vi "Link Blob To Lines.vi"(1 "Lines Calibrated":T3(array[cluster]), 2 "Blob Array":T2(array[cluster])) -> (0 "TargetArray":T1(array[cluster]))   [LabVIEW 2011]
uses:
  <vilib>/Analysis/geometry.llb/Point in Polygon Position.ctl
  <vilib>/Analysis/geometry.llb/Point in Polygon (Scalar).vi
  <vilib>/vision/NI_Vision_Development_Module.lvlib
  <vilib>/Analysis/NI_AAL_Geometry.lvlib
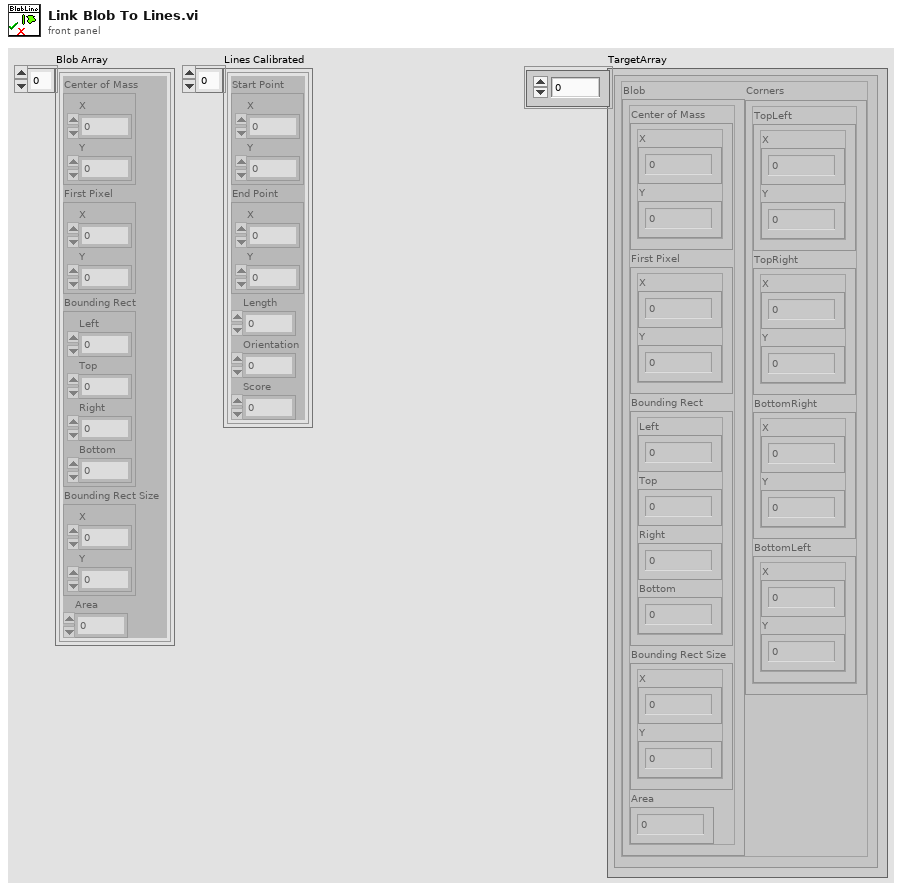
[diagram p1: front panel]
types:
  T1 = cluster{"Blob":cluster{"Center of Mass":cluster{"X":dbl, "Y":dbl}, "First Pixel":cluster{"X":dbl, "Y":dbl}, "Bounding Rect":cluster{"Left":dbl, "Top":dbl, "Right":dbl, "Bottom":dbl}, "Bounding Rect Size":cluster{"X":dbl, "Y":dbl}, "Area":dbl}, "Corners":cluster{"TopLeft":cluster{"X":dbl, "Y":dbl}, "TopRight":cluster{"X":dbl, "Y":dbl}, "BottomRight":cluster{"X":dbl, "Y":dbl}, "BottomLeft":cluster{"X":dbl, "Y":dbl}}}[]
  T2 = cluster{"Center of Mass":cluster{"X":dbl, "Y":dbl}, "First Pixel":cluster{"X":dbl, "Y":dbl}, "Bounding Rect":cluster{"Left":dbl, "Top":dbl, "Right":dbl, "Bottom":dbl}, "Bounding Rect Size":cluster{"X":dbl, "Y":dbl}, "Area":dbl}[]
  T3 = cluster{"Start Point":cluster{"X":sgl, "Y":sgl}, "End Point":cluster{"X":sgl, "Y":sgl}, "Length":dbl, "Orientation":dbl, "Score":dbl}[]
  T4 = cluster{"Blob":cluster{"Center of Mass":cluster{"X":dbl, "Y":dbl}, "First Pixel":cluster{"X":dbl, "Y":dbl}, "Bounding Rect":cluster{"Left":dbl, "Top":dbl, "Right":dbl, "Bottom":dbl}, "Bounding Rect Size":cluster{"X":dbl, "Y":dbl}, "Area":dbl}, "Lines":cluster{"Start Point":cluster{"X":sgl, "Y":sgl}, "End Point":cluster{"X":sgl, "Y":sgl}, "Length":dbl, "Orientation":dbl, "Score":dbl}[]}[]
  T5 = cluster{"Blob":cluster{"Center of Mass":cluster{"X":dbl, "Y":dbl}, "First Pixel":cluster{"X":dbl, "Y":dbl}, "Bounding Rect":cluster{"Left":dbl, "Top":dbl, "Right":dbl, "Bottom":dbl}, "Bounding Rect Size":cluster{"X":dbl, "Y":dbl}, "Area":dbl}, "Lines":cluster{"Start Point":cluster{"X":sgl, "Y":sgl}, "End Point":cluster{"X":sgl, "Y":sgl}, "Length":dbl, "Orientation":dbl, "Score":dbl}[]}
  T6 = typedef "NI_AAL_Geometry.lvlib/Point in Polygon Position.ctl" = u16
  T7 = cluster{"Point 1":cluster{"X":sgl, "Y":sgl}, "Point 2":cluster{"X":sgl, "Y":sgl}}
  T8 = cluster{"[0]":cluster{"X":dbl, "Y":dbl}, "[1]":cluster{"X":dbl, "Y":dbl}, "[2]":cluster{"X":dbl, "Y":dbl}, "[3]":cluster{"X":dbl, "Y":dbl}}
  T9 = cluster{"Center of Mass":cluster{"X":dbl, "Y":dbl}, "First Pixel":cluster{"X":dbl, "Y":dbl}, "Bounding Rect":cluster{"Left":dbl, "Top":dbl, "Right":dbl, "Bottom":dbl}, "Bounding Rect Size":cluster{"X":dbl, "Y":dbl}, "Area":dbl}
  T10 = cluster{"Start Point":cluster{"X":sgl, "Y":sgl}, "End Point":cluster{"X":sgl, "Y":sgl}, "Length":dbl, "Orientation":dbl, "Score":dbl}
  T11 = cluster{"Blob":cluster{"Center of Mass":cluster{"X":dbl, "Y":dbl}, "First Pixel":cluster{"X":dbl, "Y":dbl}, "Bounding Rect":cluster{"Left":dbl, "Top":dbl, "Right":dbl, "Bottom":dbl}, "Bounding Rect Size":cluster{"X":dbl, "Y":dbl}, "Area":dbl}, "cluster":cluster{"[0]":cluster{"X":dbl, "Y":dbl}, "[1]":cluster{"X":dbl, "Y":dbl}, "[2]":cluster{"X":dbl, "Y":dbl}, "[3]":cluster{"X":dbl, "Y":dbl}}}
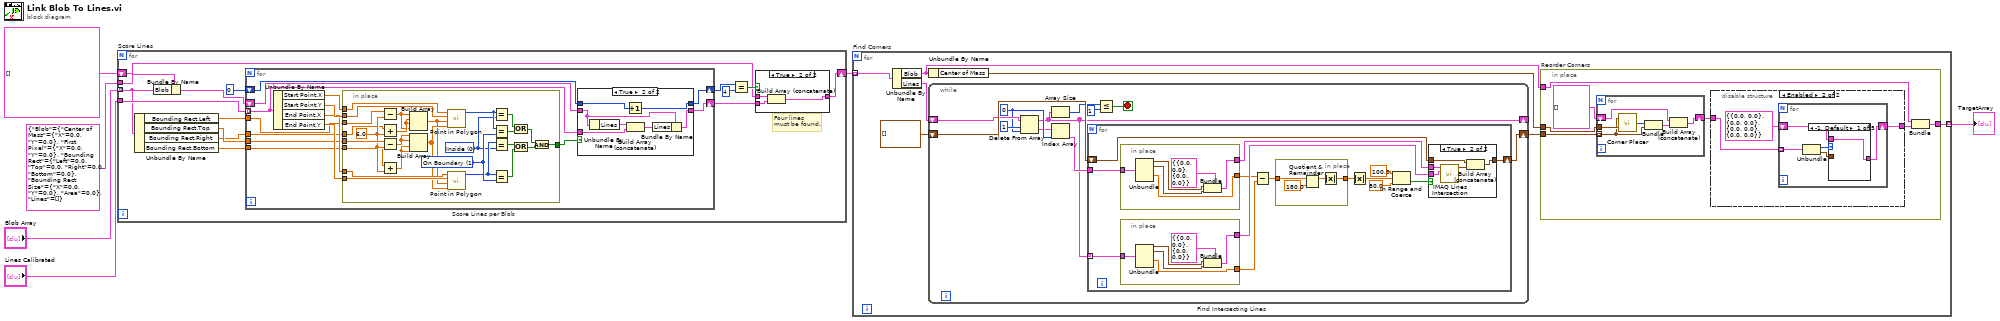
[diagram p0: block diagram]
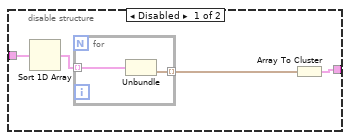
[diagram p3: hidden frame]
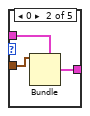
[diagram p4: hidden frame]
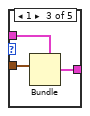
[diagram p5: hidden frame]
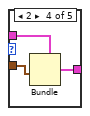
[diagram p6: hidden frame]
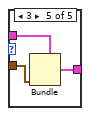
[diagram p7: hidden frame]
diagram:
  n1 = for "Score Lines" {
    tunnel: "Blob Array" -> [w15] mode=indexing
    tunnel: "Lines Calibrated" -> [w21]
    tunnel: T5 {"Blob"={"Center of Mass"={"X"=0.0, "Y"=0.0}, "First Pixel"={"X"=0.0, "Y"=0.0}, "Bounding Rect"={"Left"=0.0, "Top"=0.0, "Right"=0.0, "Bottom"=0.0}, "Bounding Rect Size"={"X"=0.0, "Y"=0.0}, "Area"=0.0}, "Lines"=[]} -> [w16]
    shift-right: [w9] -> w2
    shift-left: T4 [] -> [w8]
    # "Four lines\nmust be found."
    n2 = Unbundle By Name(w15) -> ("Bounding Rect.Left"=w20:dbl, "Bounding Rect.Top"=w19:dbl, "Bounding Rect.Right"=w18:dbl, "Bounding Rect.Bottom"=w17:dbl)
    n3 = Bundle By Name(cluster=w16, "Blob"=w15) -> (w14:T5)
    n4 = for "Score Lines per Blob" {
      tunnel: w21 -> [w32] mode=indexing
      tunnel: w20 -> [w31]
      tunnel: w19 -> [w30]
      tunnel: w18 -> [w28]
      tunnel: w17 -> [w29]
      shift-right: [w33] -> w7
      shift-left: w14 -> [w34]
      shift-right: [w27] -> w11
      shift-left: 0 -> [w26]
      n5 = Unbundle By Name(w32) -> ("Start Point.X"=w39:sgl, "Start Point.Y"=w38:sgl, "End Point.X"=w37:sgl, "End Point.Y"=w36:sgl)
      n6 = in-place {
        in-place-border: w39 -> [w56]
        in-place-border: w38 -> [w55]
        in-place-border: w37 -> [w54]
        in-place-border: w36 -> [w53]
        in-place-border: [w65] -> w35
        in-place-border: w31 -> [w64]
        in-place-border: w30 -> [w63]
        in-place-border: w29 -> [w61]
        in-place-border: w28 -> [w60]
        w47 = T6 1 items=["Inside", "On Boundary", "Outside"] ("y")
        w42 = T6 0 items=["Inside", "On Boundary", "Outside"] ("position")
        w62 = 6.0 ("y")
        n7 = Subtract(x=w64, y=w62) -> (x-y=w52:dbl)
        n8 = Add(x=w60, y=w62) -> (x+y=w59:dbl)
        n9 = Subtract(x=w63, y=w62) -> (x-y=w58:dbl)
        n10 = Add(x=w61, y=w62) -> (x+y=w57:dbl)
        n11 = Build Array(w52, w59, w59, w52) -> (w40:dbl[])
        n12 = Build Array(w58, w58, w57, w57) -> (w41:dbl[])
        n13 = call-poly <vilib>:"Point in Polygon.vi"("Polygon Y"=w41, "Polygon X"=w40, "y"=w55, "x"=w56) -> ("position"=w46:T6)  [unwired: 6 in, 1 out]
        n14 = call-poly <vilib>:"Point in Polygon.vi"("Polygon Y"=w41, "Polygon X"=w40, "y"=w53, "x"=w54) -> ("position"=w43:T6)  [unwired: 6 in, 1 out]
        n15 = Equal?(x=w46, y=w42) -> (x = y?=w48:bool)
        n16 = Equal?(x=w46, y=w47) -> (x = y?=w49:bool)
        n17 = Equal?(x=w43, y=w42) -> (x = y?=w44:bool)
        n18 = Equal?(x=w43, y=w47) -> (x = y?=w45:bool)
        n19 = Or(x=w48, y=w49) -> (x .or. y?=w51:bool)
        n20 = Or(x=w44, y=w45) -> (x .or. y?=w50:bool)
        n21 = And(x=w51, y=w50) -> (x .and. y?=w65:bool)
      }
      n22 = case shown="True" w35 {
        tunnel: [w67 w72] -> w33
        tunnel: w34 -> [w67 w74]
        tunnel: w32 -> [_ w73]
        tunnel: [w66 w68] -> w27
        tunnel: w26 -> [w66 w69]
        frame False {
        }
        frame True {
          n23 = Unbundle By Name(w74) -> ("Lines"=w71:T3)
          n24 = Increment(x=w69) -> (x+1=w68:i32)
          n25 = Build Array (concatenate)(w71, w73) -> (w70:T3)
          n26 = Bundle By Name(cluster=w74, "Lines"=w70) -> (w72:T5)
        }
      }
    }
    n27 = Equal?(x=w11, y=4) -> (x = y?=w12:bool)
    n28 = case shown="True" w12 {
      tunnel: [w22 w24] -> w9
      tunnel: w8 -> [w22 w25]
      tunnel: w7 -> [_ w23]
      frame False {
      }
      frame True {
        n29 = Build Array (concatenate)(w25, w23) -> (w24:T4)
      }
    }
  }
  n30 = for "Find Corners" {
    tunnel: w2 -> [w81] mode=indexing
    tunnel: [w77] -> w4 mode=indexing
    n31 = Unbundle By Name(w81) -> ("Blob"=w75:T9, "Lines"=w80:T3)
    n32 = Unbundle By Name(w75) -> ("Center of Mass"=w76:cluster{"X":dbl, "Y":dbl})
    n33 = while "Find Intersecting Lines" {
      shift-right: [w91] -> w78
      shift-left: cluster{"X":dbl, "Y":dbl}[] [] -> [w92]
      shift-right: [w83] -> _
      shift-left: w80 -> [w90]
      stop <- w82 stop-if-true
      w88 = 0 ("index")
      n34 = Delete From Array(array=w90, length=1, index=w88) -> (deleted portion=w87:T3, array with subset deleted=w83:T3)
      n35 = Array Size(array=w83) -> (size(s)=w85:i32)
      n36 = Index Array(array=w87, index=w88) -> (element=w86:T10)
      n37 = for {
        tunnel: w86 -> [w106]
        shift-right: [w97] -> w91
        shift-left: w92 -> [w98]
        tunnel: w83 -> [w93] mode=indexing
        n38 = in-place {
          in-place-border: w106 -> [w128]
          in-place-border: [w125] -> w105
          in-place-border: [w123] -> w103
          n39 = Unbundle(w128) -> ("Start Point"=w126:cluster{"X":sgl, "Y":sgl}, "End Point"=w127:cluster{"X":sgl, "Y":sgl}, "Orientation"=w123:dbl)  [unwired: 2 out]
          n40 = Bundle(cluster=T7 {"Point 1"={"X"=0.0, "Y"=0.0}, "Point 2"={"X"=0.0, "Y"=0.0}} ("Line 2"), "Point 1"=w126, "Point 2"=w127) -> (w125:T7)
        }
        n41 = in-place {
          in-place-border: w93 -> [w122]
          in-place-border: [w119] -> w104
          in-place-border: [w117] -> w102
          n42 = Unbundle(w122) -> ("Start Point"=w120:cluster{"X":sgl, "Y":sgl}, "End Point"=w121:cluster{"X":sgl, "Y":sgl}, "Orientation"=w117:dbl)  [unwired: 2 out]
          n43 = Bundle(cluster=T7 {"Point 1"={"X"=0.0, "Y"=0.0}, "Point 2"={"X"=0.0, "Y"=0.0}} ("Line 2"), "Point 1"=w120, "Point 2"=w121) -> (w119:T7)
        }
        n44 = Subtract(x=w103, y=w102) -> (x-y=w94:dbl)
        n45 = in-place {
          in-place-border: w94 -> [w108]
          in-place-border: [w107] -> w96
          n46 = Quotient & Remainder(x=w108, y=180.0) -> (x-y*floor(x/y)=w109:dbl)  [unwired: 1 out]
          n47 = Absolute Value(x=w109) -> (abs(x)=w107:dbl)
        }
        n48 = Absolute Value(x=w96) -> (abs(x)=w95:dbl)
        n49 = In Range and Coerce(upper limit=100.0, x=w95, lower limit=80.0) -> (In Range?=w99:bool)  [unwired: 1 out]
        n50 = case shown="True" w99 {
          tunnel: w105 -> [_ w116]
          tunnel: w104 -> [_ w115]
          tunnel: w98 -> [w111 w114]
          tunnel: [w111 w113] -> w97
          frame False {
          }
          frame True {
            n51 = call "IMAQ Lines Intersection"("Line 2"=w115, "Line 1"=w116) -> ("Intersection Point"=w112:cluster{"X":sgl, "Y":sgl})  [unwired: 7 in, 2 out]
            n52 = Build Array (concatenate)(w114, w112) -> (w113:cluster{"X":dbl, "Y":dbl}[])
          }
        }
      }
      n53 = Less Or Equal?(x=w85, y=1) -> (x <= y?=w82:bool)
    }
    n54 = in-place "Reorder Corners" {
      in-place-border: w78 -> [w135]
      in-place-border: [w133] -> w77
      in-place-border: w75 -> [w132]
      in-place-border: w76 -> [w131]
      n55 = for {
        tunnel: w135 -> [w166] mode=indexing
        tunnel: w131 -> [w168]
        shift-right: [w164] -> w129
        shift-left: cluster{"Index":i8, cluster{"X":dbl, "Y":dbl}}[] [] -> [w163]
        n56 = call "Corner Placer.vi"("Center of Mass"=w168, "Point"=w166) -> ("Index"=w167:i8)
        n57 = Bundle("Index"=w167, w166) -> (w165:cluster{"Index":i8, cluster{"X":dbl, "Y":dbl}})  [unwired: 1 in]
        n58 = Build Array (concatenate)(w163, w165) -> (w164:cluster{"Index":i8, cluster{"X":dbl, "Y":dbl}}[])
      }
      n59 = disable-structure shown="Enabled" {
        disable-tunnel: [w139 w142] -> w134
        disable-tunnel: w129 -> [w136 w143]
        frame Disabled {
          n60 = Sort 1D Array(array=w136) -> (sorted array=w138:cluster{"Index":i8, cluster{"X":dbl, "Y":dbl}}[])
          n61 = for {
            tunnel: w138 -> [w141] mode=indexing
            tunnel: [w140] -> w137 mode=indexing
            n62 = Unbundle(w141) -> (w140:cluster{"X":dbl, "Y":dbl})  [unwired: 1 out]
          }
          n63 = Array To Cluster(array=w137) -> (cluster=w139:T8)
        }
        frame Enabled {
          n64 = for {
            shift-right: [w145] -> w142
            shift-left: T8 {"[0]"={"X"=0.0, "Y"=0.0}, "[1]"={"X"=0.0, "Y"=0.0}, "[2]"={"X"=0.0, "Y"=0.0}, "[3]"={"X"=0.0, "Y"=0.0}} ("cluster") -> [w146]
            tunnel: w143 -> [w149] mode=indexing
            n65 = Unbundle(w149) -> ("Index"=w148:i8, w147:cluster{"X":dbl, "Y":dbl})
            n66 = case shown="-1, Default" w148 {
              tunnel: w147 -> [_ w151 w154 w157 w162]
              tunnel: w146 -> [w150 w153 w155 w159 w161]
              tunnel: [w150 w152 w156 w158 w160] -> w145
              frame -1, Default {
              }
              frame 0 {
                n67 = Bundle(cluster=w153, "[0]"=w151) -> (w152:T8)  [unwired: 3 in]
              }
              frame 1 {
                n68 = Bundle(cluster=w155, "[1]"=w154) -> (w156:T8)  [unwired: 3 in]
              }
              frame 2 {
                n69 = Bundle(cluster=w159, "[2]"=w157) -> (w158:T8)  [unwired: 3 in]
              }
              frame 3 {
                n70 = Bundle(cluster=w161, "[3]"=w162) -> (w160:T8)  [unwired: 3 in]
              }
            }
          }
        }
      }
      n71 = Bundle("Blob"=w132, "cluster"=w134) -> (w133:T11)  [unwired: 1 in]
    }
  }
  "TargetArray" <- w4
